vi "Query Keyboard.vi"(8 "error in (no error)":errorcluster, 11 "Stop?":bool) -> (0 "error out":errorcluster, 2 "element":T1(ring))   [LabVIEW 2013]
uses:
  <vilib>/Utility/inputDevices.llb/closeKeyboard.vi
  <vilib>/Utility/inputDevices.llb/keyboardAcquire.vi
panel:
  out "Keys Pressed":T2(array[ring])
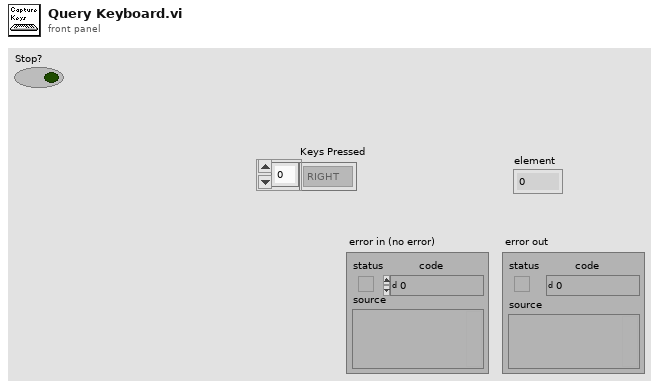
[diagram p1: front panel]
types:
  T1 = enum16{"0", "1", "2", "3", "4", "5", "6", "7", "8", "9", "A", "B", "C", "D", "E", "F", "G", "H", "I", "J", "K", "L", "M", "N", "O", "P", "Q", "R", "S", "T", "U", "V", "W", "X", "Y", "Z", "F1", "F2", "F3", "F4", "F5", "F6", "F7", "F8", "F9", "F10", "F11", "F12", "F13", "F14", "F15", "ADD", "BACK", "BACKSLASH", "CAPITAL", "COMMA", "DECIMAL", "DELETE", "DIVIDE", "DOWN", "END", "EQUALS", "ESCAPE", "GRAVE (`)", "HOME", "INSERT", "LBRACKET", "LCONTROL", "LEFT", "L ALT", "LSHIFT", "LWIN", "MINUS", "MULTIPLY", "NEXT", "NUMLOCK", "NUMPAD_0", "NUMPAD_1", "NUMPAD_2", "NUMPAD_3", "NUMPAD_4", "NUMPAD_5", "NUMPAD_6", "NUMPAD_7", "NUMPAD_8", "NUMPAD_9", "PAUSE", "PERIOD", "PRIOR (PG UP)", "RBRACKET", "RCONTROL", "RETURN", "RIGHT", "R ALT", "RSHIFT", "RWIN", "SCROLL", "SEMICOLON", "SLASH", "SPACE", "SUBTRACT", "TAB", "UP", "ENTER (num pad)", "' (quote)"}
  T2 = enum16{"0", "1", "2", "3", "4", "5", "6", "7", "8", "9", "A", "B", "C", "D", "E", "F", "G", "H", "I", "J", "K", "L", "M", "N", "O", "P", "Q", "R", "S", "T", "U", "V", "W", "X", "Y", "Z", "F1", "F2", "F3", "F4", "F5", "F6", "F7", "F8", "F9", "F10", "F11", "F12", "F13", "F14", "F15", "ADD", "BACK", "BACKSLASH", "CAPITAL", "COMMA", "DECIMAL", "DELETE", "DIVIDE", "DOWN", "END", "EQUALS", "ESCAPE", "GRAVE (`)", "HOME", "INSERT", "LBRACKET", "LCONTROL", "LEFT", "L ALT", "LSHIFT", "LWIN", "MINUS", "MULTIPLY", "NEXT", "NUMLOCK", "NUMPAD_0", "NUMPAD_1", "NUMPAD_2", "NUMPAD_3", "NUMPAD_4", "NUMPAD_5", "NUMPAD_6", "NUMPAD_7", "NUMPAD_8", "NUMPAD_9", "PAUSE", "PERIOD", "PRIOR (PG UP)", "RBRACKET", "RCONTROL", "RETURN", "RIGHT", "R ALT", "RSHIFT", "RWIN", "SCROLL", "SEMICOLON", "SLASH", "SPACE", "SUBTRACT", "TAB", "UP", "ENTER (num pad)", "' (quote)"}[]
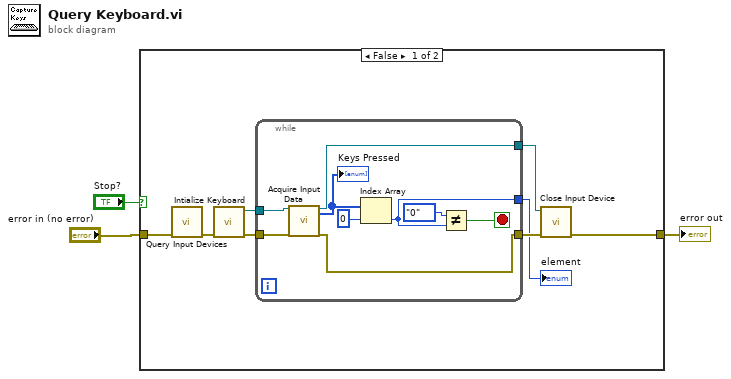
[diagram p0: block diagram]
diagram:
  n1 = case shown="False" "Stop?" {
    tunnel: "error in (no error)" -> [w4 w21]
    tunnel: [w7 w21] -> w2
    frame False {
      n2 = call <vilib>:"Query Input Devices.vi"("error in (no error)"=w4) -> ("error out"=w10:errorcluster)  [unwired: 7 in, 3 out]
      n3 = call <vilib>:"Intialize Keyboard.vi"("error in (no error)"=w10) -> ("error out"=w5:errorcluster, "device ID"=w11:refnum<k1>)  [unwired: 9 in]
      n4 = while {
        tunnel: w11 -> [w20]
        tunnel: w5 -> [w19]
        tunnel: [w18] -> w9
        tunnel: [w12] -> w8
        tunnel: [w13] -> w6
        stop <- w15 stop-if-true
        n5 = call-poly <vilib>:"Acquire Input Data.vi"("device ID"=w20, "error in (no error)"=w19) -> ("device ID"=w18:refnum<k1>, "keys pressed"=w14:T2, "error out"=w12:errorcluster)  [unwired: 15 in]
        "Keys Pressed" <- w14
        n6 = Index Array(array=w14, index=0) -> (element=w13:T1)
        n7 = Not Equal?(x=T1."0", y=w13) -> (x != y?=w15:bool)
      }
      "element" <- w6
      n8 = call-poly <vilib>:"Close Input Device.vi"("error in (no error)"=w8, "device ID"=w9) -> ("error out"=w7:errorcluster)  [unwired: 8 out]
    }
    frame True {
    }
  }
  "error out" <- w2
